vi "Create.vi"(8 "error in (no error)":errorcluster, 10 "group configuration":T1={"core"={"name"="Group", "direction"=enum."Tx", "cycle timing"={"priority"=100, "decimation"=1, "offset"=0}, "timeout behavior"=enum."Increment Late Count"}, "component settings"=[], "transfers"=[]} {"transfers"."channels"."core"."string offset" format="%d bytes"}, 11 "Group Configuration in":refnum<class "Group Configuration.lvclass">) -> (0 "error out":errorcluster, 3 "Group Configuration out":refnum<class "Group Configuration.lvclass">)   [LabVIEW 2017, in "DSF Core.lvlib" / "Group Configuration.lvclass"]
uses:
  Group Configuration.lvclass
  C:/Git/DSF/Core/Classes/Configuration/Runtime/Runtime Configuration.lvclass
  Typedefs/DSF Engine Transfer Group Configuration.ctl
  Typedefs/DSF Core Group Configuration.ctl
  Typedefs/DSF Direction.ctl
  Typedefs/DSF Timing Info.ctl
  Typedefs/DSF Timeout Behavior.ctl
  Typedefs/DSF Settings Info.ctl
  Typedefs/DSF Version Info.ctl
  Typedefs/DSF Engine Transfer Configuration.ctl
  Typedefs/DSF Core Transfer Configuration.ctl
  Typedefs/DSF Engine Channel Configuration.ctl
  Typedefs/DSF Core Channel Configuration.ctl
  Typedefs/DSF Data Type.ctl
  Group Configuration.lvclass/Group Configuration.ctl
  Transfer/Transfer Configuration.lvclass
  Runtime/Runtime Configuration.lvclass
  DSF Core.lvlib
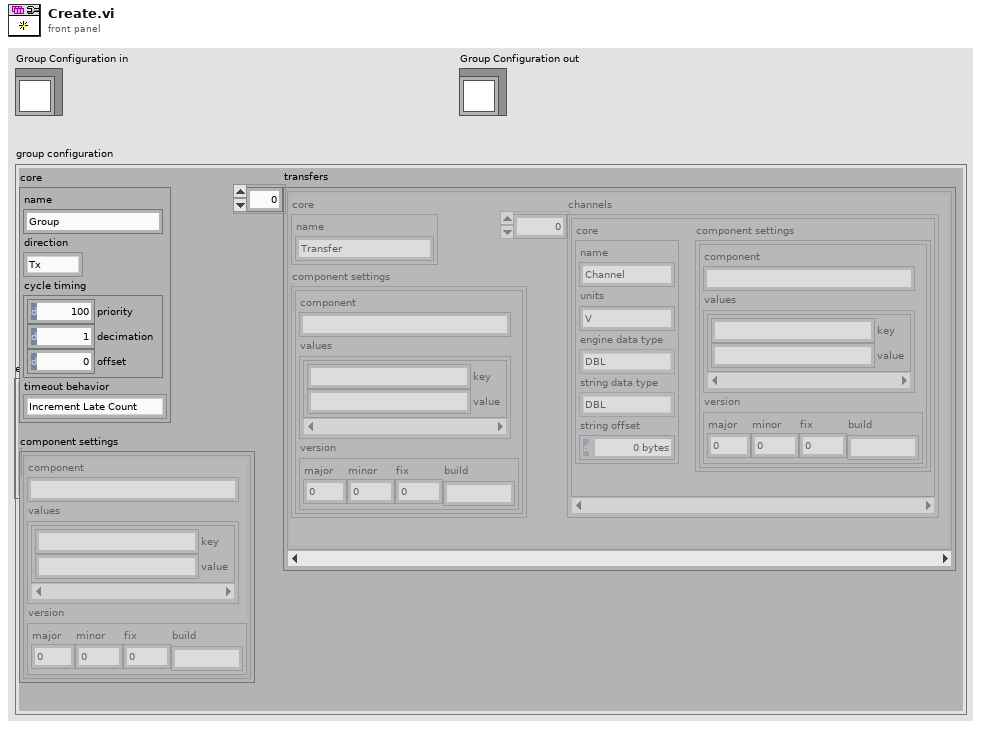
[diagram p1: front panel]
types:
  T1 = typedef "DSF Core.lvlib/DSF Engine Transfer Group Configuration.ctl" = cluster{"core":T2, "component settings":T6[], "transfers":T8[]}
  T2 = typedef "DSF Core.lvlib/DSF Core Group Configuration.ctl" = cluster{"name":string, "direction":T3, "cycle timing":T4, "timeout behavior":T5}
  T3 = typedef "DSF Core.lvlib/DSF Direction.ctl" = enum8{"Tx", "Rx"}
  T4 = typedef "DSF Core.lvlib/DSF Timing Info.ctl" = cluster{"priority":u64, "decimation":u64, "offset":u64}
  T5 = typedef "DSF Core.lvlib/DSF Timeout Behavior.ctl" = enum8{"Increment Late Count", "Throw Error"}
  T6 = typedef "DSF Core.lvlib/DSF Settings Info.ctl" = cluster{"component":string, "values":cluster{"key":string, "value":string}[], "version":T7}
  T7 = typedef "DSF Core.lvlib/DSF Version Info.ctl" = cluster{"major":u32, "minor":u32, "fix":u32, "build":string}
  T8 = typedef "DSF Core.lvlib/DSF Engine Transfer Configuration.ctl" = cluster{"core":T9, "component settings":T6[], "channels":T10[]}
  T9 = typedef "DSF Core.lvlib/DSF Core Transfer Configuration.ctl" = cluster{"name":string}
  T10 = typedef "DSF Core.lvlib/DSF Engine Channel Configuration.ctl" = cluster{"core":T11, "component settings":T6[]}
  T11 = typedef "DSF Core.lvlib/DSF Core Channel Configuration.ctl" = cluster{"name":string, "units":string, "engine data type":T12, "string data type":T12, "string offset":u64}
  T12 = typedef "DSF Core.lvlib/DSF Data Type.ctl" = enum8{"Bool", "SGL", "DBL", "I8", "I16", "I32", "I64", "U8", "U16", "U32", "U64"}
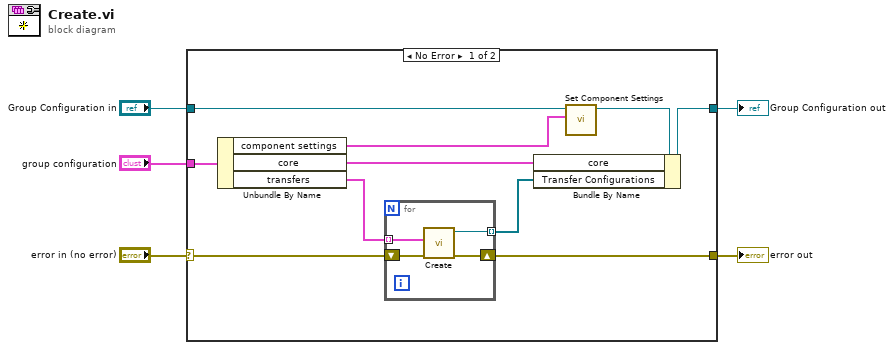
[diagram p0: block diagram]
diagram:
  n1 = case shown="No Error" "error in (no error)" {
    selector: "error in (no error)" -> [w12 w21]
    tunnel: [w11 w21] -> w4
    tunnel: [w14 w20] -> w2
    tunnel: "Group Configuration in" -> [w8 w20]
    tunnel: "group configuration" -> [w15 _]
    frame No Error {
      n2 = Unbundle By Name(w15) -> ("component settings"=w6:T6[], "core"=w13:T2, "transfers"=w9:T8[])
      n3 = for {
        shift-right: [w18] -> w11
        shift-left: w12 -> [w19]
        tunnel: [w17] -> w10 mode=indexing
        tunnel: w9 -> [w16] mode=indexing
        n4 = call "Create.vi"("error in (no error)"=w19, "transfer configuration"=w16) -> ("error out"=w18:errorcluster, "Transfer Configuration out"=w17:refnum<class "Transfer Configuration.lvclass">)  [unwired: 8 in]
      }
      n5 = call "Set Component Settings.vi"("component settings"=w6, "Runtime Configuration in"=w8) -> ("Runtime Configuration out"=w7:refnum<class "Group Configuration.lvclass">)  [unwired: 8 in, 1 out]
      n6 = Bundle By Name(cluster=w7, "core"=w13, "Transfer Configurations"=w10) -> (w14:refnum<class "Group Configuration.lvclass">)
    }
    frame Error {
    }
  }
  "error out" <- w4
  "Group Configuration out" <- w2
